vi "Scripting Constants.vi"() -> ()   [LabVIEW 2017, in "Switch Scripting.lvlib"]
doc: "Use this Global VI to access the GUIDs assigned to the page resources of the Custom Device."
uses:
  Switch Scripting.lvlib
panel:
  in  "Tab Control":T1(tab)=enum."SLSC Switch Constants"
  in  "SLSC Switch:CD:GUID":string="5e47c8de-3ec6-490b-8897-5526d4aea756"
  in  "RAF:CD:GUID":string="4e591626-626d-4903-9a6e-1f2a7b879f4d"
  in  "RAF:Channel:Descriptions":string="Descriptions"
  in  "RAF:State:Description":string="_Description"
  in  "RAF:State:DefaultValue":i32
  in  "RAF:State:DefaultName":string="Default"
  in  "RAF:Routes":string="Routes"
  in  "RAF:Aliases":string="Aliases"
  in  "RAF:Channel:Connections":string="Connections"
  in  "RAF:Name":string="Routing and Faulting Custom Device"
  in  "SLSC Switch:Endpoint Configuration":string="Endpoint Configuration"
  in  "SLSC Switch:Capabilities":string="Capabilities "
  in  "SLSC Switch:Capabilities Version":string="Capabilities Version"
  in  "SLSC Switch:Topology":string="Topology "
  in  "SLSC Switch:Resource":string="Resource "
  in  "SLSC Switch:Model":string="Model"
  in  "Compiled.Settings":string="Compiled.Settings"
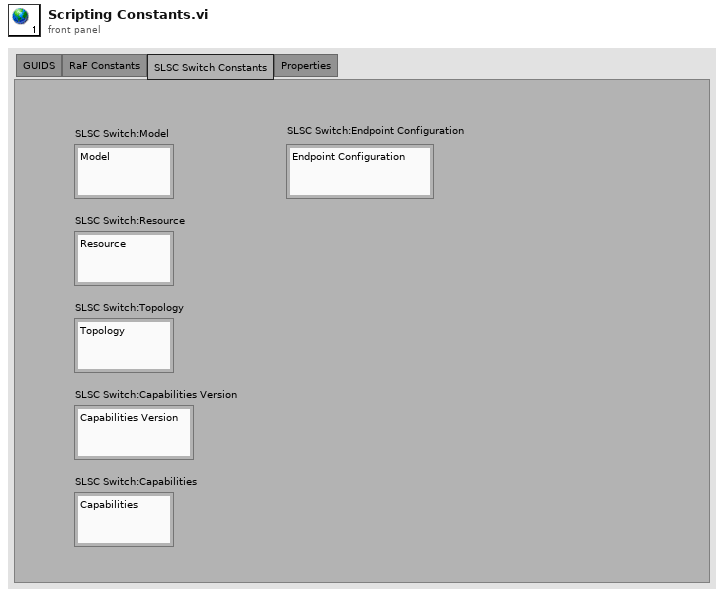
[diagram p1: front panel]
types:
  T1 = enum32{"GUIDS", "RaF Constants", "SLSC Switch Constants", "Properties"}
diagram:
